vi "淡出.vi"(8 "错误输入（无错误）":errorcluster, 11 "引用输入":refnum<vi>) -> (0 "error out":errorcluster caption="错误输出", 3 "引用输出":refnum<vi>)   [LabVIEW 8.6, in "窗口操作.lvlib"]
doc: "<B>引用输入：</B>需要改变窗口的引用\n<B>引用输出：</B>需要改变窗口的引用输出\n\n编写者 ：曾嘉康\n编写时间：2014/12/12"
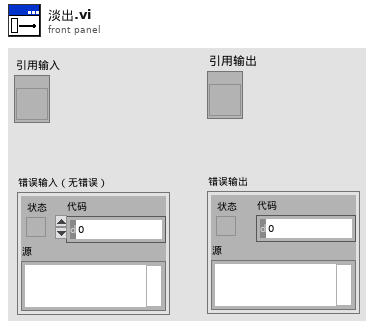
[diagram p1: front panel]
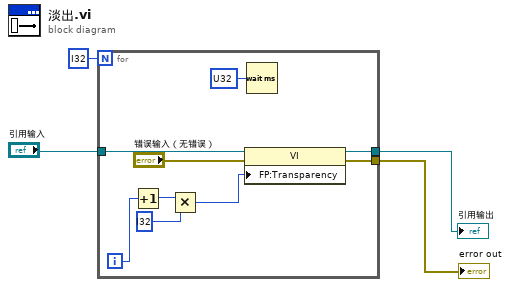
[diagram p0: block diagram]
diagram:
  n1 = for {
    N: i32 ? -> [_]
    tunnel: [w9] -> w2
    tunnel: "引用输入" -> [w7]
    tunnel: [w5] -> w1
    i -> [w13]
    n2 = Increment(x=w13) -> (x+1=w12:i32)
    n3 = Multiply(x=w12, y=i32 ?) -> (x*y=w10:i32)
    n4 = property class="VI"(reference=w7, error in="错误输入（无错误）", "FP:Transparency"=w10) -> (reference out=w5:refnum<vi>, error out=w9:errorcluster)
    n5 = Wait (ms)(milliseconds to wait=u32 ? ("等待时间（毫秒）")) -> ()  [unwired: 1 out]
  }
  "error out" <- w2
  "引用输出" <- w1
